vi "tsdb_get_flexray_db_ecu_properties_by_index.vi"(8 "error in (no error)":errorcluster caption="错误输入（无错误）", 9 "FECUIndex":i32, 10 "FDBIndex":i32, 11 "路径输入":path=path "D:/Program Files (x86)/TOSUN/TSMaster/bin/TSMaster.dll") -> (0 "error out":errorcluster caption="错误输出", 1 "TDBECUProperties":T1, 2 "function return":i32, 3 "路径输出":path)   [LabVIEW 2014]
doc: "Function Introduction\nRetrieve ECU properties of specified LIN database through index\nCall location\ninput parameter \nAvalue: The returned attribute data structure, please search for the definition in the TSMaster header\nReturn value\n==0: Execution successful\nOther values: Query error code"
uses:
  Typedef/TDBECUProperties.ctl
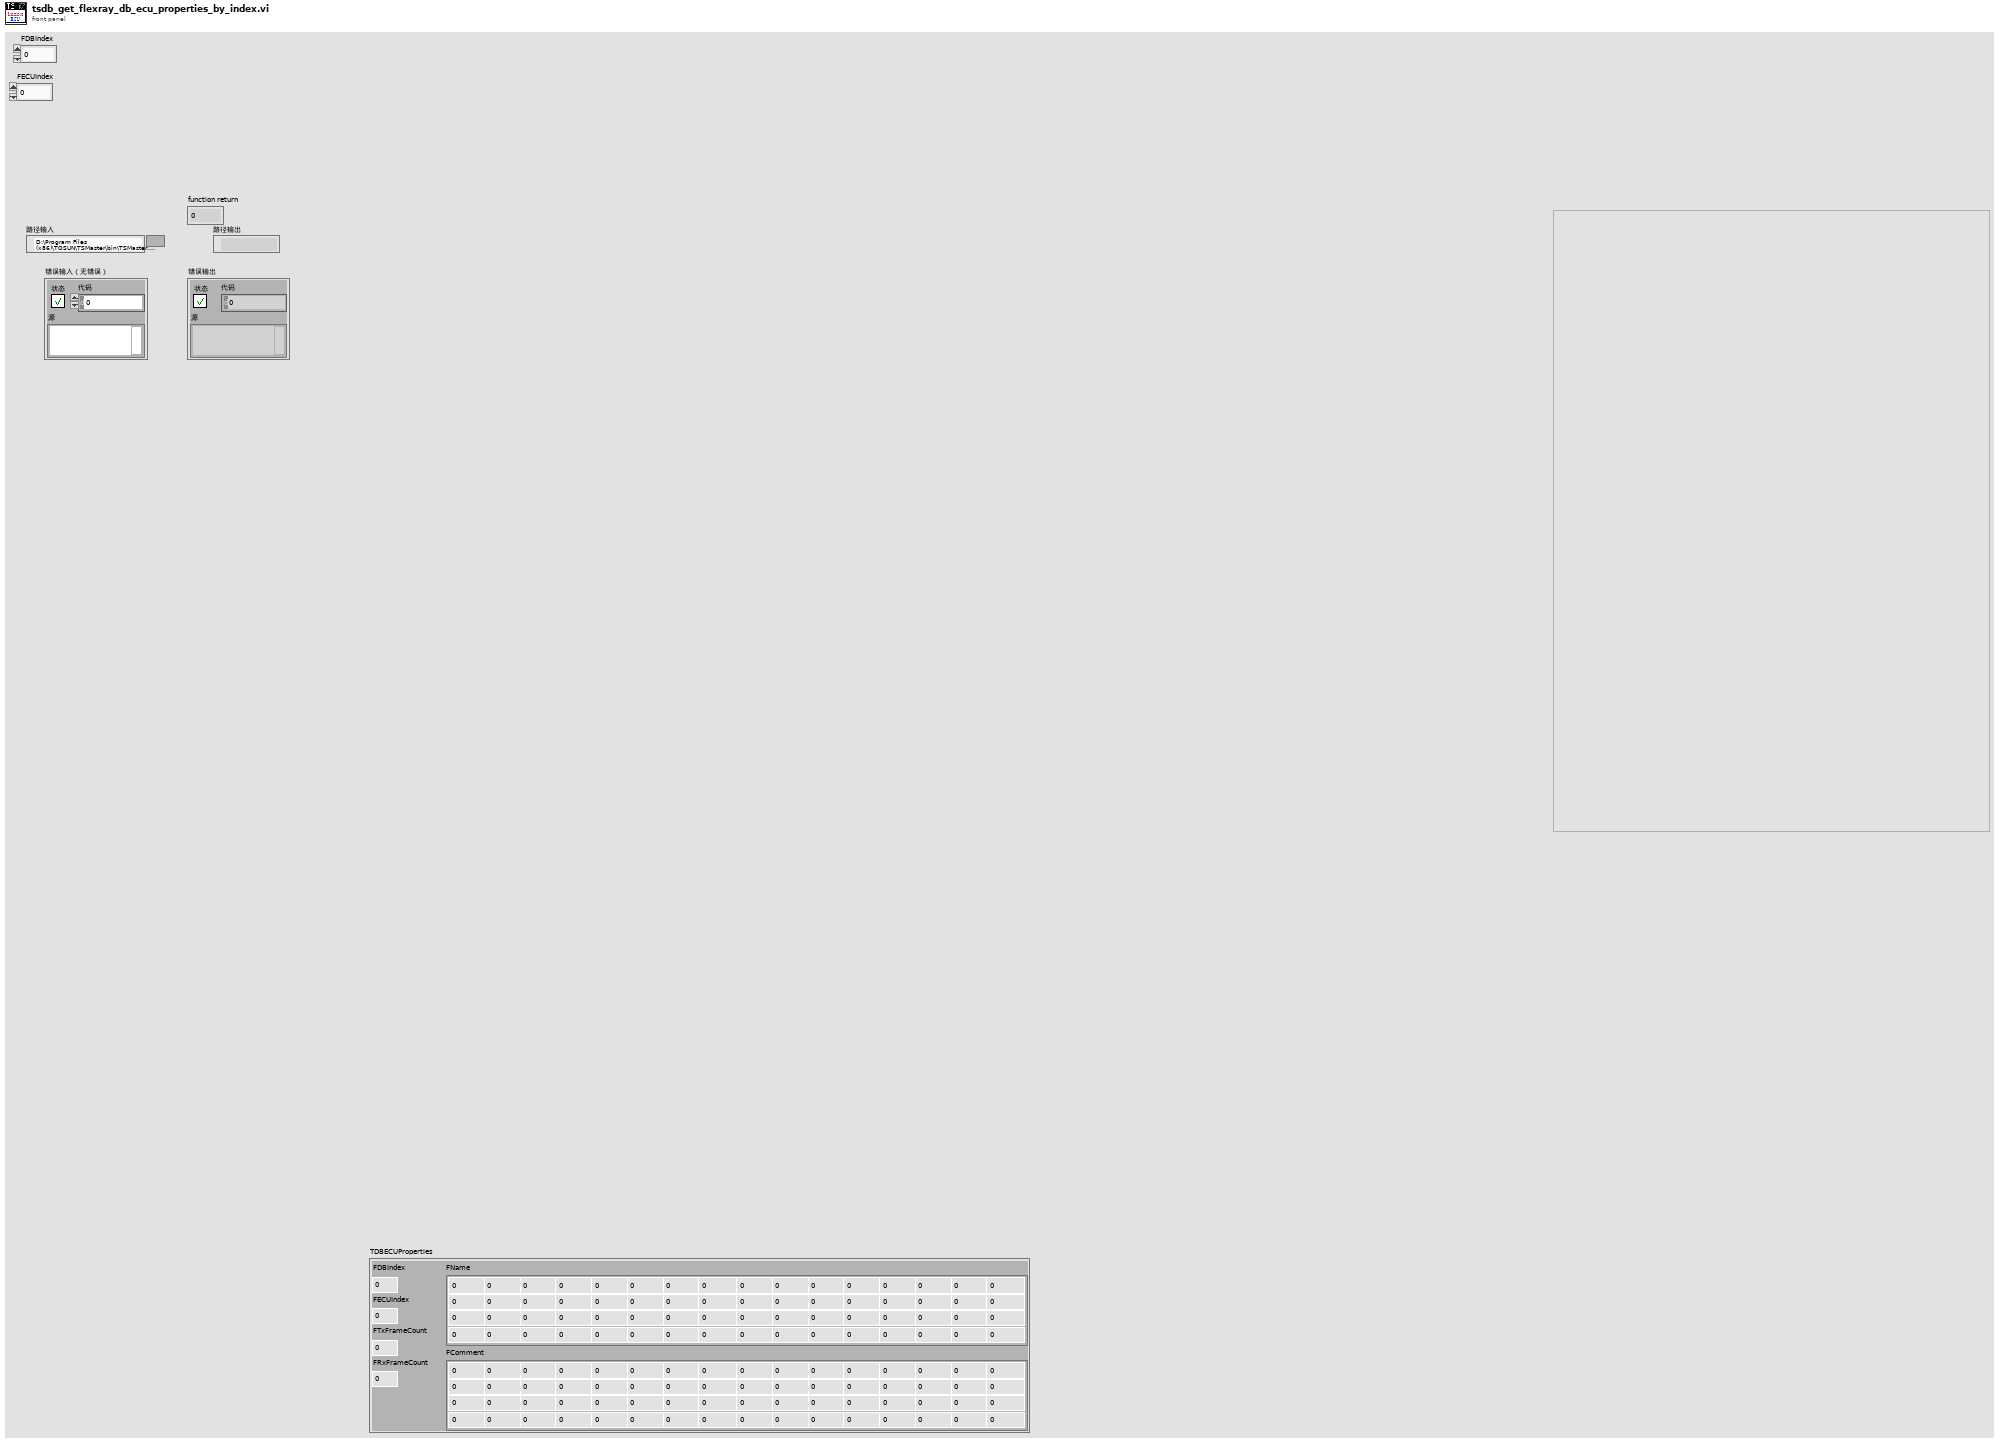
[diagram p1: front panel]
types:
  T1 = typedef "TDBECUProperties.ctl" = cluster{"FDBIndex":i32, "FECUIndex":i32, "FTxFrameCount":i32, "FRxFrameCount":i32, "FName":cluster{"数值":u64, "数值 2":u64, "数值 3":u64, "数值 4":u64, "数值 5":u64, "数值 6":u64, "数值 7":u64, "数值 8":u64, "数值 9":u64, "数值 10":u64, "数值 11":u64, "数值 12":u64, "数值 13":u64, "数值 14":u64, "数值 15":u64, "数值 16":u64, "数值 17":u64, "数值 18":u64, "数值 19":u64, "数值 20":u64, "数值 21":u64, "数值 22":u64, "数值 23":u64, "数值 24":u64, "数值 25":u64, "数值 26":u64, "数值 27":u64, "数值 28":u64, "数值 29":u64, "数值 30":u64, "数值 31":u64, "数值 32":u64, "数值 33":u64, "数值 34":u64, "数值 35":u64, "数值 36":u64, "数值 37":u64, "数值 38":u64, "数值 39":u64, "数值 40":u64, "数值 41":u64, "数值 42":u64, "数值 43":u64, "数值 44":u64, "数值 45":u64, "数值 46":u64, "数值 47":u64, "数值 48":u64, "数值 49":u64, "数值 50":u64, "数值 51":u64, "数值 52":u64, "数值 53":u64, "数值 54":u64, "数值 55":u64, "数值 56":u64, "数值 57":u64, "数值 58":u64, "数值 59":u64, "数值 60":u64, "数值 61":u64, "数值 62":u64, "数值 63":u64, "数值 64":u64}, "FComment":cluster{"数值":u64, "数值 2":u64, "数值 3":u64, "数值 4":u64, "数值 5":u64, "数值 6":u64, "数值 7":u64, "数值 8":u64, "数值 9":u64, "数值 10":u64, "数值 11":u64, "数值 12":u64, "数值 13":u64, "数值 14":u64, "数值 15":u64, "数值 16":u64, "数值 17":u64, "数值 18":u64, "数值 19":u64, "数值 20":u64, "数值 21":u64, "数值 22":u64, "数值 23":u64, "数值 24":u64, "数值 25":u64, "数值 26":u64, "数值 27":u64, "数值 28":u64, "数值 29":u64, "数值 30":u64, "数值 31":u64, "数值 32":u64, "数值 33":u64, "数值 34":u64, "数值 35":u64, "数值 36":u64, "数值 37":u64, "数值 38":u64, "数值 39":u64, "数值 40":u64, "数值 41":u64, "数值 42":u64, "数值 43":u64, "数值 44":u64, "数值 45":u64, "数值 46":u64, "数值 47":u64, "数值 48":u64, "数值 49":u64, "数值 50":u64, "数值 51":u64, "数值 52":u64, "数值 53":u64, "数值 54":u64, "数值 55":u64, "数值 56":u64, "数值 57":u64, "数值 58":u64, "数值 59":u64, "数值 60":u64, "数值 61":u64, "数值 62":u64, "数值 63":u64, "数值 64":u64}}
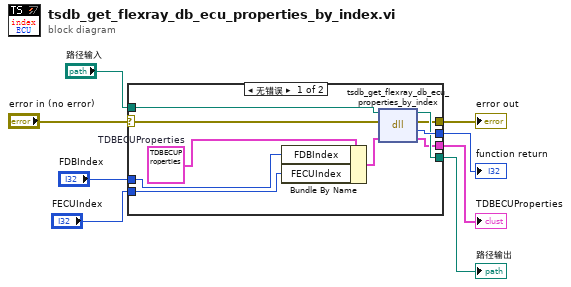
[diagram p0: block diagram]
diagram:
  n1 = case shown="无错误" "error in (no error)" {
    selector: "error in (no error)" -> [w9 w20]
    tunnel: [w18 _] -> w8
    tunnel: "路径输入" -> [w17 w19]
    tunnel: [w16 w19] -> w6
    tunnel: [w15 w20] -> w5
    tunnel: [w14 _] -> w4
    tunnel: "FECUIndex" -> [w11 _]
    tunnel: "FDBIndex" -> [w10 _]
    frame No Error {
      w13 = T1 {"FDBIndex"=0, "FECUIndex"=0, "FTxFrameCount"=0, "FRxFrameCount"=0, "FName"={"数值"=0, "数值 2"=0, "数值 3"=0, "数值 4"=0, "数值 5"=0, "数值 6"=0, "数值 7"=0, "数值 8"=0, "数值 9"=0, "数值 10"=0, "数值 11"=0, "数值 12"=0, "数值 13"=0, "数值 14"=0, "数值 15"=0, "数值 16"=0, "数值 17"=0, "数值 18"=0, "数值 19"=0, "数值 20"=0, "数值 21"=0, "数值 22"=0, "数值 23"=0, "数值 24"=0, "数值 25"=0, "数值 26"=0, "数值 27"=0, "数值 28"=0, "数值 29"=0, "数值 30"=0, "数值 31"=0, "数值 32"=0, "数值 33"=0, "数值 34"=0, "数值 35"=0, "数值 36"=0, "数值 37"=0, "数值 38"=0, "数值 39"=0, "数值 40"=0, "数值 41"=0, "数值 42"=0, "数值 43"=0, "数值 44"=0, "数值 45"=0, "数值 46"=0, "数值 47"=0, "数值 48"=0, "数值 49"=0, "数值 50"=0, "数值 51"=0, "数值 52"=0, "数值 53"=0, "数值 54"=0, "数值 55"=0, "数值 56"=0, "数值 57"=0, "数值 58"=0, "数值 59"=0, "数值 60"=0, "数值 61"=0, "数值 62"=0, "数值 63"=0, "数值 64"=0}, "FComment"={"数值"=0, "数值 2"=0, "数值 3"=0, "数值 4"=0, "数值 5"=0, "数值 6"=0, "数值 7"=0, "数值 8"=0, "数值 9"=0, "数值 10"=0, "数值 11"=0, "数值 12"=0, "数值 13"=0, "数值 14"=0, "数值 15"=0, "数值 16"=0, "数值 17"=0, "数值 18"=0, "数值 19"=0, "数值 20"=0, "数值 21"=0, "数值 22"=0, "数值 23"=0, "数值 24"=0, "数值 25"=0, "数值 26"=0, "数值 27"=0, "数值 28"=0, "数值 29"=0, "数值 30"=0, "数值 31"=0, "数值 32"=0, "数值 33"=0, "数值 34"=0, "数值 35"=0, "数值 36"=0, "数值 37"=0, "数值 38"=0, "数值 39"=0, "数值 40"=0, "数值 41"=0, "数值 42"=0, "数值 43"=0, "数值 44"=0, "数值 45"=0, "数值 46"=0, "数值 47"=0, "数值 48"=0, "数值 49"=0, "数值 50"=0, "数值 51"=0, "数值 52"=0, "数值 53"=0, "数值 54"=0, "数值 55"=0, "数值 56"=0, "数值 57"=0, "数值 58"=0, "数值 59"=0, "数值 60"=0, "数值 61"=0, "数值 62"=0, "数值 63"=0, "数值 64"=0}}  # TDBECUProperties
      n2 = Bundle By Name(cluster=w13, "FDBIndex"=w10, "FECUIndex"=w11) -> (w12:T1)
      n3 = dll-call lib="D:/Program Files (x86)/TOSUN/TSMaster/bin/TSMaster.dll" fn="tsdb_get_flexray_db_ecu_properties_by_index"(path in=w17, error in=w9, "Avalue"=w12) -> (path out=w16:path, error out=w15:errorcluster, "返回类型"=w18:i32, "Avalue"=w14:T1)  [unwired: 1 in]
    }
    frame Error {
    }
  }
  "function return" <- w8
  "error out" <- w5
  "路径输出" <- w6
  "TDBECUProperties" <- w4
